vi "Launch Configured Nested.vi"(8 "error in (no error)":errorcluster, 11 "Task in":refnum<class "Task.lvclass">) -> (0 "error out":errorcluster, 3 "Task out":refnum<class "Task.lvclass">)   [LabVIEW 2020, in "Volatus.lvlib" / "Task.lvclass"]
uses:
  Task.lvclass
  Task.lvclass/Task.ctl
  VolatusConfig/VolatusConfig.lvlib
  VolatusConfig/Meta Type.ctl
  lv-cdm/CDM-Config/Config Manager/Config Manager.lvclass
  VolatusConfig/Task/Task.lvclass
  Volatus.lvlib
  lv-cdm/CDM-Config/Config Element/Config Element.lvclass
  VolatusConfig/VolatusConfigElement/VolatusConfigElement.lvclass
  C:/dev/lv20CE/relink/lv-volatus/VolatusConfig/VolatusConfigElement/VolatusConfigElement.lvclass
  C:/dev/lv20CE/relink/lv-volatus/VolatusConfig/Task/Task.lvclass
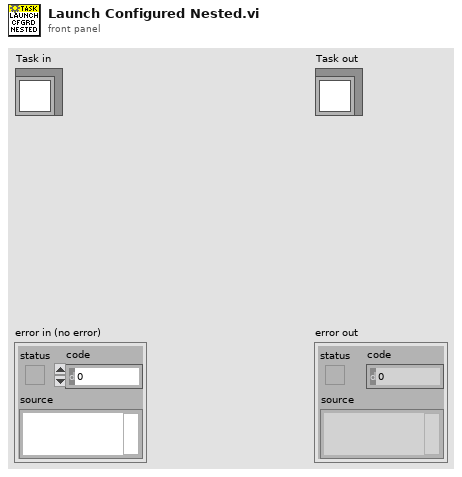
[diagram p1: front panel]
types:
  T1 = typedef "VolatusConfig.lvlib/Meta Type.ctl" = enum16{"UNKNOWN", "VL_System", "VL_Cluster", "VL_Node", "VL_Task", "VL_Group", "VL_Channel", "VL_Task_List", "VL_Scaling", "VL_Sensor", "VL_Sensor_List", "VL_Scale"}
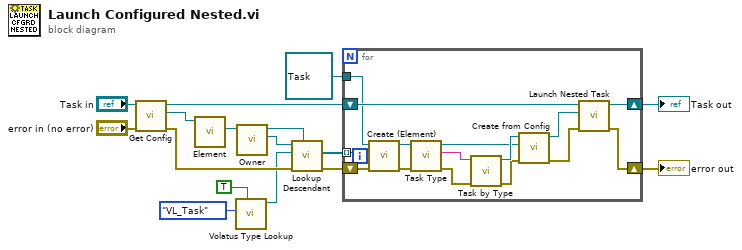
[diagram p0: block diagram]
diagram:
  n1 = call "Get Config.vi"("error in (no error)"="error in (no error)", "Task in"="Task in") -> ("error out"=w16:errorcluster, "Config"=w13:refnum<class "Task.lvclass">, "Task out"=w6:refnum<class "Task.lvclass">)  [unwired: 7 in]
  n2 = call "Element.vi"("VolatusConfigElement in"=w13) -> ("Element"=w12:refnum<class "Config Element.lvclass">)  [unwired: 9 in, 1 out]
  n3 = call "Volatus Type Lookup.vi"("Don't Recurse Past Match (F)"=TRUE, "Meta Type"=Meta_Type."VL_Task") -> ("Config Lookup out"=w8:refnum<class "Config Lookup.lvclass">)  [unwired: 8 in, 1 out]
  n4 = call "Owner.vi"("Config Element in"=w12) -> ("Owner"=w9:refnum<class "Config Manager.lvclass">, "Config Element out"=w7:refnum<class "Config Element.lvclass">)  [unwired: 8 in, 1 out]
  n5 = call "Lookup Descendant.vi"("Start (Root)"=w7, "error in (no error)"=w16, "Lookup"=w8, "Config Manager in"=w9) -> ("error out"=w5:errorcluster, "Descendants"=w3:refnum<class "Config Element.lvclass">[])  [unwired: 5 in, 1 out]
  n6 = for {
    shift-right: [w22] -> w2
    shift-left: w6 -> [w23]
    shift-right: [w21] -> w4
    shift-left: w5 -> [w31]
    tunnel: w3 -> [w20] mode=indexing
    tunnel: refnum<class "Task.lvclass"> refnum ("VolatusConfig.lvlib:Task.lvclass") -> [w17]
    n7 = call "Create (Element).vi"("error in (no error)"=w31, "Element"=w20, "VolatusConfigElement in"=w17) -> ("error out"=w18:errorcluster, "VolatusConfigElement in"=w19:refnum<class "Task.lvclass">)  [unwired: 7 in]
    n8 = call "Task Type.vi"("error in (no error)"=w18, "Task in"=w19) -> ("error out"=w30:errorcluster, "Task Type"=w29:string, "Task out"=w26:refnum<class "Task.lvclass">)  [unwired: 7 in]
    n9 = call "Task by Type.vi"("error in (no error)"=w30, "Task Type"=w29) -> ("error out"=w27:errorcluster, "Task"=w28:refnum<class "Task.lvclass">)  [unwired: 8 in]
    n10 = call "Create from Config.vi"("error in (no error)"=w27, "Config"=w26, "Task in"=w28) -> ("error out"=w24:errorcluster, "Task out"=w25:refnum<class "Task.lvclass">)  [unwired: 7 in]
    n11 = call "Launch Nested Task.vi"("error in (no error)"=w24, "Nested Task"=w25, "Task in"=w23) -> ("error out"=w21:errorcluster, "Task out"=w22:refnum<class "Task.lvclass">)  [unwired: 6 in, 1 out]
  }
  "error out" <- w4
  "Task out" <- w2
